vi "Read Job.vi"(11 "Jobber in":refnum<class "Jobber.lvclass">) -> (2 "Job.lvclass":refnum<class "Job.lvclass">)   [LabVIEW 2014, in "Jobber.lvlib" / "Jobber.lvclass"]
uses:
  Jobber.lvclass
  Classes/Job/Job.lvclass
  Jobber.lvclass/Jobber.ctl
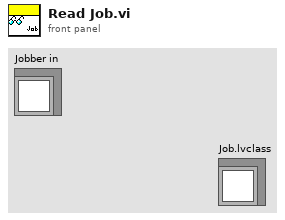
[diagram p1: front panel]
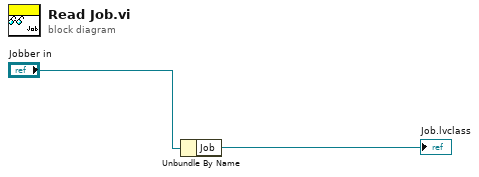
[diagram p0: block diagram]
diagram:
  n1 = Unbundle By Name("Jobber in") -> ("Job"=→"Job.lvclass":refnum<class "Job.lvclass">)
